vi "Convex Hull 2D (GiftWrap) example.vi"() -> ()   [LabVIEW 2016]
panel:
  in  "Random start pts":bool=TRUE
  in  "Npts random":i32=32
  in  "Points":sgl[][](array[numeric])=[[0.0, 0.0, 0.0], [10.0, 0.0, 0.0], [10.0, 10.0, 0.0], [0.0, 10.0, 0.0], [50.0, 50.0, 0.0], [60.0, 50.0, 0.0], [60.0, 60.0, 0.0], [50.0, 60.0, 0.0]]
  out "Visualisation":cluster{sgl[], sgl[]}[](graph)
  # "PN 17/03/2015,\n      11/08/2017"
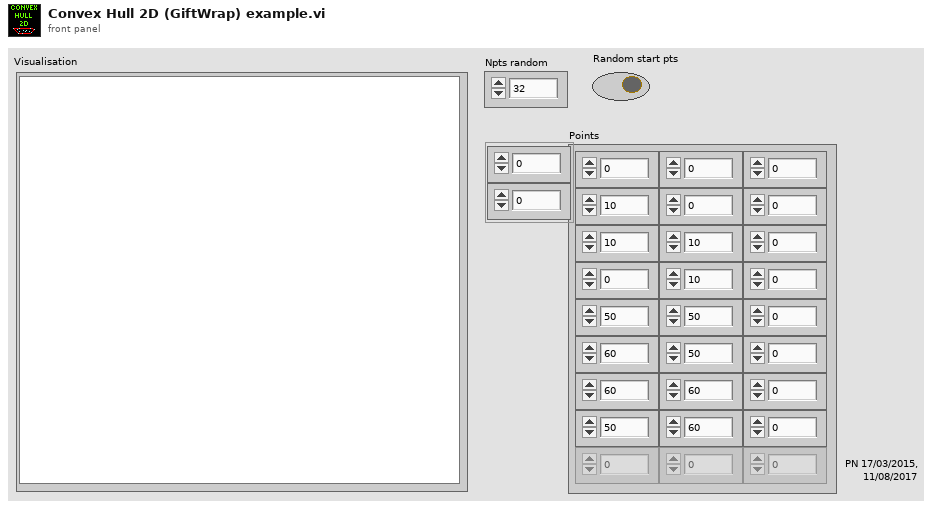
[diagram p1: front panel]
types:
  T1 = typedef "Edge, indexed.ctl" = cluster{"V0":sgl[], "V1":sgl[], "i0":i32, "i1":i32}
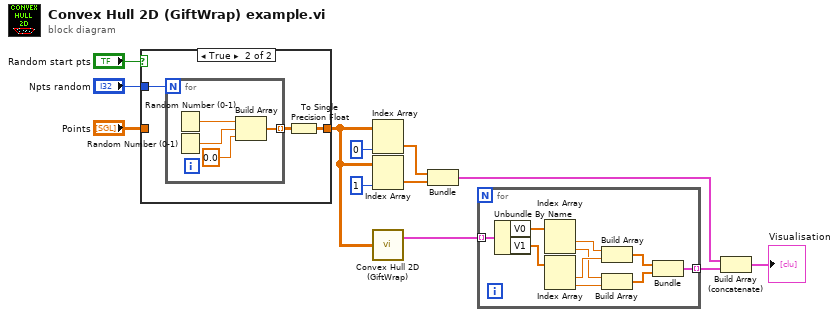
[diagram p0: block diagram]
diagram:
  n1 = case shown="True" "Random start pts" {
    tunnel: "Npts random" -> [_ w15]
    tunnel: "Points" -> [w13 _]
    tunnel: [w13 w14] -> w2
    frame False {
    }
    frame True {
      n2 = for {
        N: w15 -> [_]
        tunnel: [w17] -> w16 mode=indexing
        n3 = Random Number (0-1)() -> (number: 0 to 1=w20:dbl)
        n4 = Random Number (0-1)() -> (number: 0 to 1=w19:dbl)
        n5 = Build Array(w20, w19, 0.0 ("element")) -> (w17:dbl[])
      }
      n6 = To Single Precision Float(number=w16) -> (single precision float=w14:sgl[][])
    }
  }
  n7 = Index Array(array=w2, index (col)=0 ("disabled index (col)")) -> (element=w5:sgl[])  [unwired: 1 in]
  n8 = Index Array(array=w2, index (col)=1 ("disabled index (col)")) -> (element=w3:sgl[])  [unwired: 1 in]
  n9 = call "Convex Hull 2D (GiftWrap).vi"("Points"=w2) -> ("Convex Hull lines"=w1:T1[])  [unwired: 1 out]
  n10 = Bundle("Points"=w5, "Points"=w3) -> (w7:cluster{"Points":sgl[], "Points":sgl[]})  [unwired: 1 in]
  n11 = for {
    tunnel: [w22] -> w11 mode=indexing
    tunnel: w1 -> [w21] mode=indexing
    n12 = Unbundle By Name(w21) -> ("V0"=w24:sgl[], "V1"=w23:sgl[])
    n13 = Index Array(array=w24) -> (element #1=w30:sgl, element #2=w27:sgl)  [unwired: 2 in]
    n14 = Index Array(array=w23) -> (element #1=w28:sgl, element #2=w26:sgl)  [unwired: 2 in]
    n15 = Build Array(w30, w28) -> (w29:sgl[])
    n16 = Build Array(w27, w26) -> (w25:sgl[])
    n17 = Bundle(w29, w25) -> (w22:cluster{sgl[], sgl[]})  [unwired: 1 in]
  }
  n18 = Build Array (concatenate)(w7, w11) -> (→"Visualisation":cluster{"Points":sgl[], "Points":sgl[]}[])
